vi "construct lorentzian.vi"(10 "omega  in":dbl[](array[numeric]), 11 "lorentzian":T1={"A (VHz)"=-1.0311345636926572, "f (Hz)"=-1.0311345636926572, "G (Hz)"=-1.0311345636926572, "phi(rad)"=-1.0311345636926572, "Q"=-1.0311345636926572, "Norm  Ampl"=-1.0311345636926572, "bg (V)"=-1.0311345636926572+0.0i, "4corners"={"z (-pi/2)"=-1.0311345636926572+0.5736824521422934i, "z(inf)"=-0.5200164984937075+1.0975277942502903i, "z (pi/2)"=-1.0311345636926572+0.5736824521422934i, "z center"=-0.5136528600391839+0.580046090596817i, "z(0)"=-0.5200164984937075+1.0975277942502903i, "radius"=-1.0311345636926572}} {"bg (V)" format="%#9_9f"; "Q" format="%#9_9f"; "phi(rad)" format="%#9_9f"; "G (Hz)" format="%#9_9f"; "f (Hz)" format="%#9_9f"}) -> (2 "omega  out":dbl[](array[numeric]), 3 "z out":cdb[](array[numeric]))   [LabVIEW 2018]
uses:
  lorentzian.ctl
  circle corners.ctl
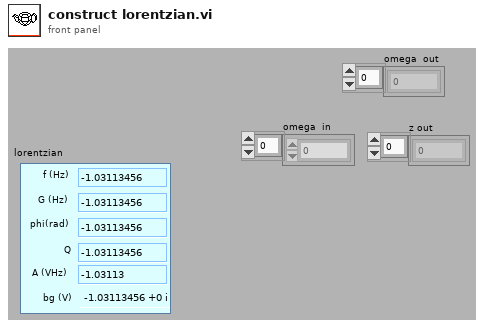
[diagram p1: front panel]
types:
  T1 = typedef "lorentzian.ctl" = cluster{"A (VHz)":dbl, "f (Hz)":dbl, "G (Hz)":dbl, "phi(rad)":dbl, "Q":dbl, "Norm  Ampl":dbl, "bg (V)":cdb, "4corners":T2}
  T2 = typedef "circle corners.ctl" = cluster{"z (-pi/2)":cdb, "z(inf)":cdb, "z (pi/2)":cdb, "z center":cdb, "z(0)":cdb, "radius":dbl}
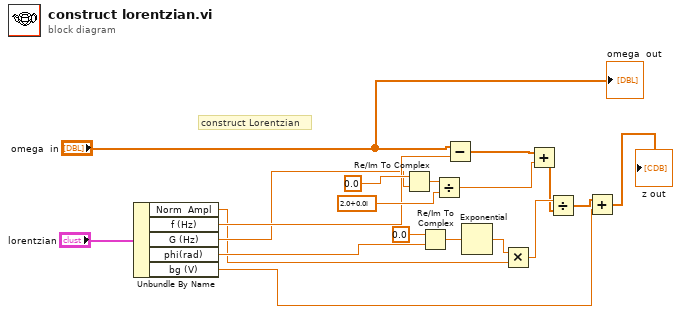
[diagram p0: block diagram]
diagram:
  # "construct Lorentzian"
  n1 = Unbundle By Name("lorentzian") -> ("Norm  Ampl"=w5:dbl, "f (Hz)"=w8:dbl, "G (Hz)"=w7:dbl, "phi(rad)"=w6:dbl, "bg (V)"=w1:cdb)
  n2 = Re/Im To Complex(1:w7, 2:0.0 ("x")) -> (0:w13:cdb)
  n3 = Re/Im To Complex(1:w6, 2:0.0 ("x")) -> (0:w18:cdb)
  n4 = Divide(x=w13, y=cdb 2.0+0.0i) -> (x/y=w11:cdb)
  n5 = Subtract(x="omega  in", y=w8) -> (x-y=w15:dbl[])
  n6 = Exponential(1:w18) -> (0:w17:cdb)
  n7 = Multiply(x=w17, y=w5) -> (x*y=w16:cdb)
  n8 = Add(x=w15, y=w11) -> (x+y=w10:cdb[])
  n9 = Divide(x=w16, y=w10) -> (x/y=w9:cdb[])
  n10 = Add(x=w9, y=w1) -> (x+y=→"z out":cdb[])
  "omega  out" <- "omega  in"
